vi "IOTEST.vi"() -> ()   [LabVIEW 2013]
uses:
  <userlib>/DAQNavi Polymorphic VI/create/DAQNavi Create Channel(DO-Digital Output).vi
  <userlib>/DAQNavi Polymorphic VI/write/DAQNavi Write (Digital U8 1Chan 1Samp).vi
panel:
  out "error out":errorcluster
  in  "error in (no error)":errorcluster
  in  "data":u8 format="%x"
  in  "physical channels":string="USB-4761,BID#0/port0"
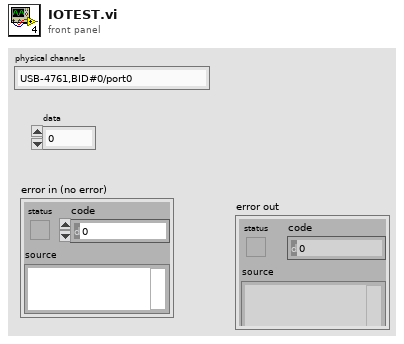
[diagram p1: front panel]
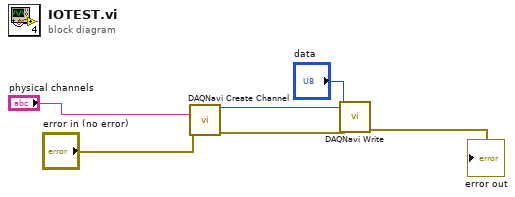
[diagram p0: block diagram]
diagram:
  n1 = call-poly <userlib>:"DAQNavi Create Channel.vi"("physical channels"="physical channels", "error in (no error)"="error in (no error)") -> ("task out"=w5:i32, "error out"=w4:errorcluster)  [unwired: 12 in]
  n2 = call-poly <userlib>:"DAQNavi Write.vi"("error in (no error)"=w4, "data"="data", "task in"=w5) -> ("error out"=→"error out":errorcluster)  [unwired: 6 in, 2 out]
